vi "LH_TailPushListNode.vi"(2 "Content":i32, 3 "InputList":refnum<class "ListHead.lvclass">) -> (1 "OutputList":refnum<class "ListHead.lvclass">)   [LabVIEW 2014, in "ListHead.lvclass"]
uses:
  ListHead.lvclass
  ListHead.lvclass/ListHead.ctl
  ListNode.lvclass
  ListNodeVirtual.lvclass
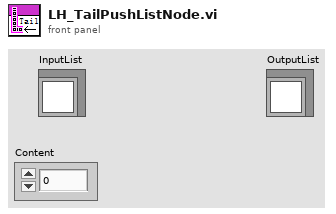
[diagram p1: front panel]
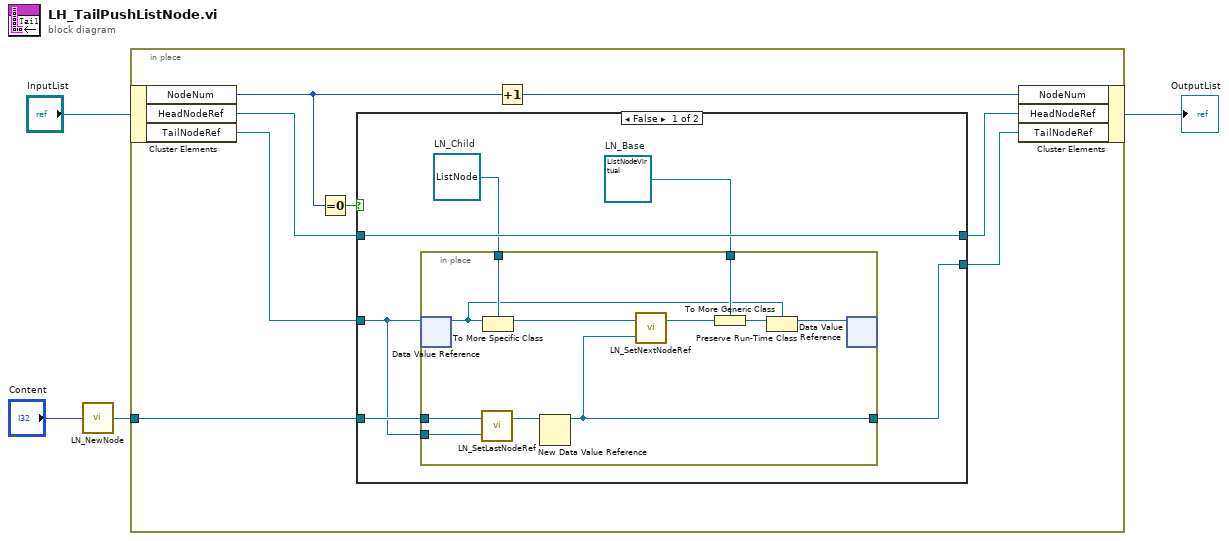
[diagram p0: block diagram]
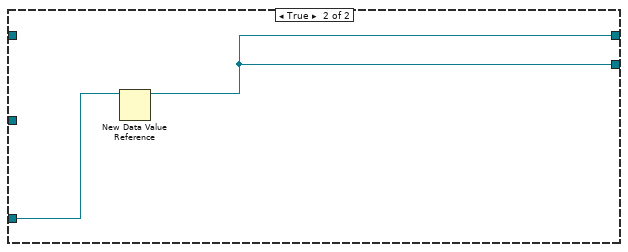
[diagram p2: hidden frame]
diagram:
  n1 = call "LN_NewNode.vi"("InputContent"="Content") -> ("OutputListNode"=w2:refnum<class "ListNode.lvclass">)
  n2 = in-place {
    in-place-border: w2 -> [w11]
    n3 = in-place-cluster #1("InputList") -> ("NodeNum"=w10:u32, "HeadNodeRef"=w8:refnum<data-value>, "TailNodeRef"=w7:refnum<data-value>)
    n4 = Equal To 0?(x=w10) -> (x = 0?=w12:bool)
    n5 = case shown="False" w12 {
      tunnel: w11 -> [w15 w31]
      tunnel: w8 -> [w18 _]
      tunnel: w7 -> [w14 _]
      tunnel: [w17 w30] -> w5
      tunnel: [w18 w30] -> w6
      frame False {
        w13 = refnum<class "ListNodeVirtual.lvclass"> refnum  # LN_Base
        w16 = refnum<class "ListNode.lvclass"> refnum  # LN_Child
        n6 = in-place {
          in-place-border: [w24] -> w17
          in-place-border: w16 -> [w29]
          in-place-border: w15 -> [w27]
          in-place-border: w14 -> [w26]
          in-place-border: w13 -> [w22]
          n7 = in-place-dvr #2(w14) -> (w20:refnum<class "ListNodeVirtual.lvclass">)  [unwired: 1 out]
          n8 = call "LN_SetLastNodeRef.vi"("InputLastNodeRef"=w26, "InputListNode"=w27) -> ("OutputListNode"=w25:refnum<class "ListNode.lvclass">)  [unwired: 1 in]
          n9 = To More Specific Class(target class=w29, reference=w20) -> (specific class reference=w28:refnum<class "ListNode.lvclass">)  [unwired: 1 in, 1 out]
          n10 = New Data Value Reference(data value=w25) -> (data value reference=w24:refnum<data-value>)  [unwired: 1 in, 1 out]
          n11 = call "LN_SetNextNodeRef.vi"("InputNextNodeRef"=w24, "InputListNode"=w28) -> ("OutputListNode"=w23:refnum<class "ListNode.lvclass">)  [unwired: 1 in]
          n12 = To More Generic Class(target class=w22, reference=w23) -> (generic class reference=w21:refnum<class "ListNodeVirtual.lvclass">)
          n13 = Preserve Run-Time Class(object in=w21, 2:w20) -> (object out=w19:refnum<class "ListNodeVirtual.lvclass">)  [unwired: 1 in, 1 out]
          n14 = in-place-dvr #2(w19) -> ()  [unwired: 2 out]
        }
      }
      frame True {
        n15 = New Data Value Reference(data value=w31) -> (data value reference=w30:refnum<data-value>)  [unwired: 1 in, 1 out]
      }
    }
    n16 = Increment(x=w10) -> (x+1=w9:u32)
    n17 = in-place-cluster #1("NodeNum"=w9, "HeadNodeRef"=w6, "TailNodeRef"=w5) -> (→"OutputList":refnum<class "ListHead.lvclass">)
  }
